vi "Mutexed Merge Errors.vi"(6 "Publish Time (Use Current Time)":timestamp, 8 "error in (no error)":errorcluster, 9 "Error or Array of Errors":variant, 10 "Datum Name":string, 11 "IModel in":refnum<class "IModel.lvclass">) -> (0 "error out":errorcluster, 3 "IModel out":refnum<class "IModel.lvclass">)   [LabVIEW 2018, in "MVA Framework.lvlib" / "IModel.lvlib" / "IModel.lvclass"]
doc: "互斥合并错误"
uses:
  IModel.lvclass
  IMediator/IMediator Messages/Publish Msg/Publish Msg.lvclass
  IObserver/IObserver/IObserver.lvclass
  IMediator/MutexedPublishRequest/MutexedPublishRequest.lvclass
  <vilib>/Utility/Data Type/NI_Data Type.lvlib
  <vilib>/ErrorRing/Error Ring.xnode
  PublicationPolicy/MergeErrorsPublication/MergeErrorsPublication.lvclass
  C:/Program Files/National Instruments/LabVIEW 2020/vi.lib/ActorFramework/Actor/Actor.lvclass
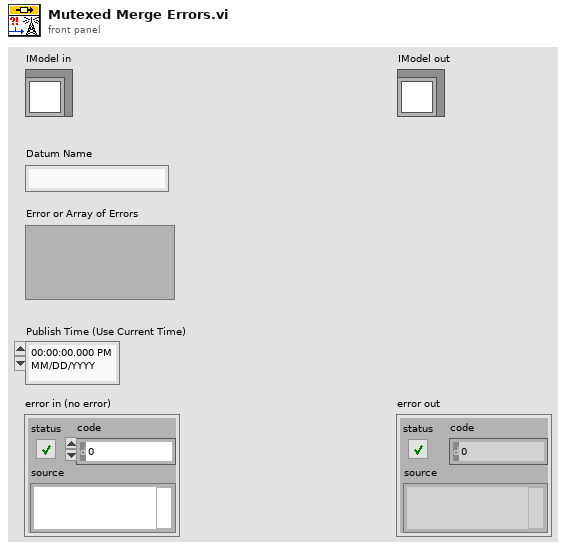
[diagram p1: front panel]
types:
  T1 = typedef "NI_Data Type.lvlib/Data Type.ctl" = enum8{"Invalid Type", "Void", "I8", "I16", "I32", "I64", "U8", "U16", "U32", "U64", "Single Float", "Double Float", "Extended Float", "Single Complex", "Double Complex", "Extended Complex", "Enum U8", "Enum U16", "Enum U32", "Enum U64", "Single Float With Unit", "Double Float With Unit", "Extended Float With Unit", "Single Complex with Unit", "Double Complex with Unit", "Extended Complex with Unit", "Boolean", "String", "Path", "Picture", "Tag", "Array", "Cluster", "Variant", "LV Variant", "Waveform", "Timestamp", "Digital Waveform", "Digital Data", "ExpressData", "Refnum", "External Data", "VI", "Poly VI", "LabVIEW Class Instance", "Fixed Point", "Set Collection", "Map Collection"}
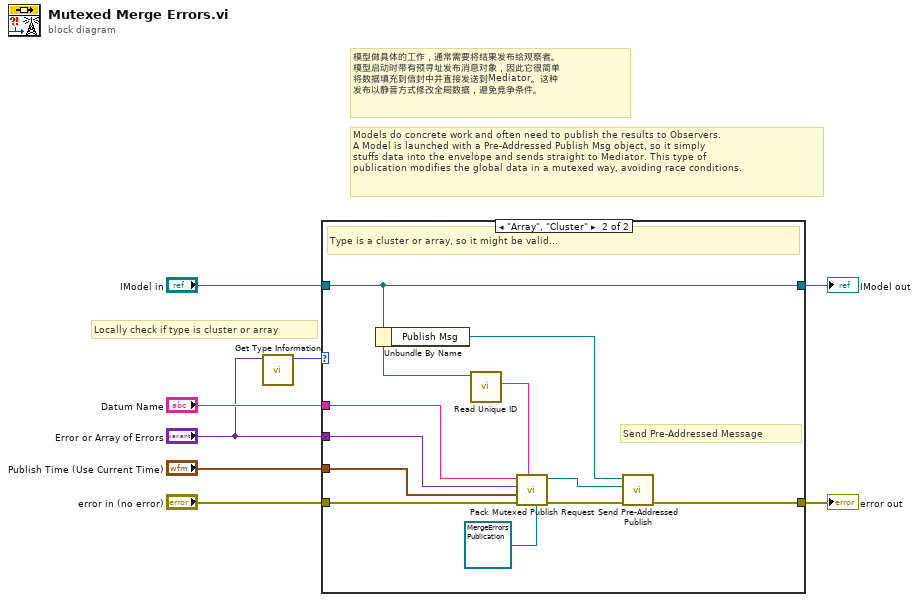
[diagram p0: block diagram]
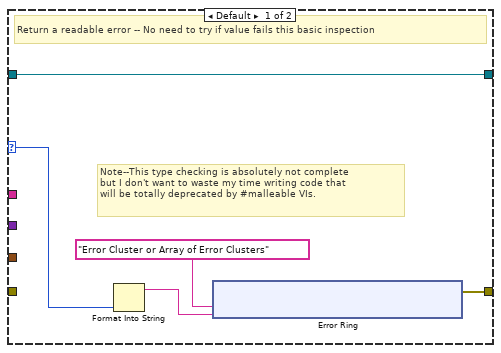
[diagram p2: hidden frame]
diagram:
  # "模型做具体的工作，通常需要将结果发布给观察者。\n模型启动时带有预寻址发布消息对象，因此它很简单\n将数据填充到信封中并直接发送到Mediator。这种\n发布以静音方式修改全局数据，避免竞争条件。"
  # "Locally check if type is cluster or array"
  # "Models do concrete work and often need to publish the results to Observers.\nA Model is launched with a Pre-Addressed Publish Msg object, so it simply\nstuffs data into the envelope and sends straight to Mediator. This type of\npublication modifies the global data in a mutexed way, avoiding race conditions."
  n1 = call <vilib>:"Get Type Information.vi"("variant"="Error or Array of Errors") -> ("type"=w1:T1)  [unwired: 6 in, 4 out]
  n2 = case shown="\"Array\", \"Cluster\"" w1 {
    selector: w1 -> [w9 _]
    tunnel: "error in (no error)" -> [_ w22]
    tunnel: [w12 w29] -> w7
    tunnel: "IModel in" -> [w13 w24]
    tunnel: "Datum Name" -> [_ w28]
    tunnel: "Error or Array of Errors" -> [_ w27]
    tunnel: "Publish Time (Use Current Time)" -> [_ w26]
    tunnel: [w13 w24] -> w3
    frame Default {
      # "Note--This type checking is absolutely not complete\nbut I don't want to waste my time writing code that\nwill be totally deprecated by #malleable VIs."
      # "Return a readable error -- No need to try if value fails this basic inspection"
      n3 = Format Into String(w9) -> (resulting string=w10:string)  [unwired: 3 in, 1 out]
      n4 = xnode "Error Ring"("参数 0"="Error Cluster or Array of Error Clusters" ("parameter 0"), "参数 1"=w10) -> ("错误输出"=w12:errorcluster)
    }
    frame "Array", "Cluster" {
      # "Send Pre-Addressed Message"
      # "Type is a cluster or array, so it might be valid..."
      n5 = Unbundle By Name(w24) -> ("Publish Msg"=w30:refnum<class "Publish Msg.lvclass">)
      n6 = call "Read Unique ID.vi"("IObserver In"=w24) -> ("Unique ID"=w23:string)  [unwired: 10 in]
      n7 = call "Pack Mutexed Publish Request.vi"("PublicationPolicy"=refnum<class "MergeErrorsPublication.lvclass"> refnum ("PublicationPolicy.lvlib:MergeErrorsPublication.lvclass"), "Publisher ID"=w23, "error in (no error)"=w22, "Publish Time (Use Current Time)"=w26, "Datum Value or Type"=w27, "Datum Name"=w28) -> ("error out"=w21:errorcluster, "MutexedPublishRequest Out"=w25:refnum<class "MutexedPublishRequest.lvclass">)  [unwired: 4 in]
      n8 = call "Send Pre-Addressed Publish.vi"("error in (no error)"=w21, "PublishRequest"=w25, "Publish Message"=w30) -> ("error out"=w29:errorcluster)  [unwired: 8 in]
    }
  }
  "IModel out" <- w3
  "error out" <- w7
